vi "Output Processing.vi"(0 "Measurements":T2, 5 "Software Flags":T1, 7 "Powerdown?":bool, 11 "error in (no error)":errorcluster) -> (4 "Measurement Results":T4, 15 "error out":errorcluster)   [LabVIEW 2024, in "devicePowerSequencerCoreLogic.lvlib"]
uses:
  devicePowerSequencerCoreLogic.lvlib
  Measurement Results.ctl
  controls/Measurements.ctl
  controls/Voltage and Current Measurements.ctl
  controls/Software Flags.ctl
  <vilib>/Utility/error.llb/Trim Whitespace One-Sided.vi
  Device Power Sequencer.lvlib
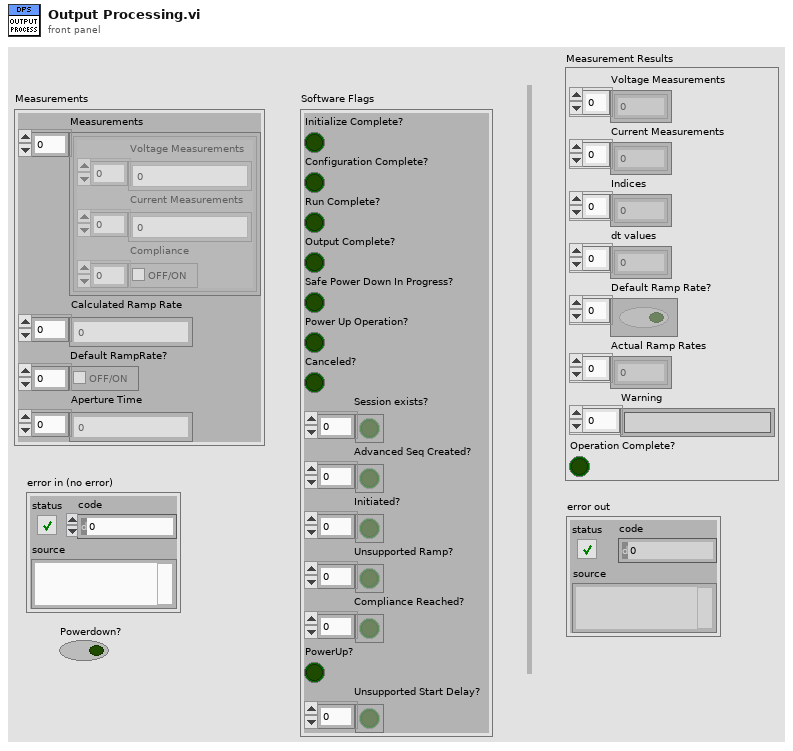
[diagram p1: front panel]
types:
  T1 = typedef "devicePowerSequencerCoreLogic.lvlib/Software Flags.ctl" = cluster{"Initialize Complete?":bool, "Configuration Complete?":bool, "Run Complete?":bool, "Output Complete?":bool, "Safe Power Down In Progress?":bool, "Power Up Operation?":bool, "Canceled?":bool, "Session exists?":bool[], "Advanced Seq Created?":bool[], "Initiated?":bool[], "Unsupported Ramp?":bool[], "Compliance Reached?":bool[], "PowerUp?":bool, "Unsupported Start Delay?":bool[]}
  T2 = typedef "devicePowerSequencerCoreLogic.lvlib/Measurements.ctl" = cluster{"Measurements":T3[], "Calculated Ramp Rate":dbl[], "Default RampRate?":bool[], "Aperture Time":dbl[]}
  T3 = typedef "devicePowerSequencerCoreLogic.lvlib/Voltage and Current Measurements.ctl" = cluster{"Voltage Measurements":dbl[], "Current Measurements":dbl[], "Compliance":bool[]}
  T4 = typedef "Device Power Sequencer.lvlib/Measurement Results.ctl" = cluster{"Voltage Measurements":dbl[], "Current Measurements":dbl[], "Indices":i32[], "dt values":dbl[], "Default Ramp Rate?":bool[], "Actual Ramp Rates":dbl[], "Warning":string[], "Operation Complete?":bool}
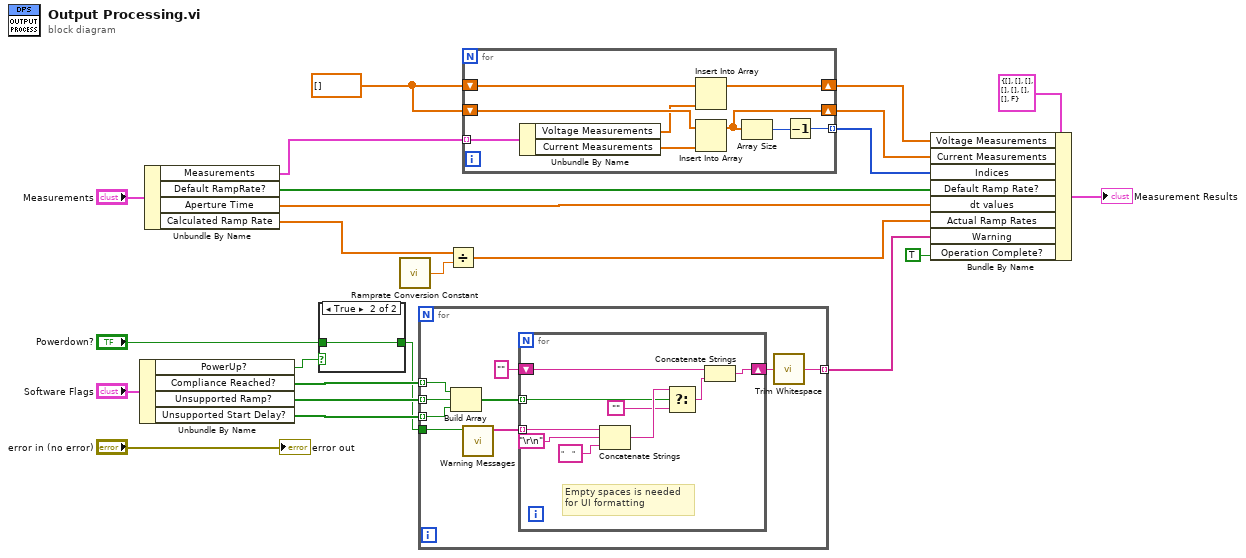
[diagram p0: block diagram]
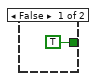
[diagram p2: hidden frame]
diagram:
  w23 = dbl[] []
  n1 = Unbundle By Name("Software Flags") -> ("PowerUp?"=w4:bool, "Compliance Reached?"=w14:bool[], "Unsupported Ramp?"=w13:bool[], "Unsupported Start Delay?"=w5:bool[])
  n2 = Unbundle By Name("Measurements") -> ("Measurements"=w6:T3[], "Default RampRate?"=w18:bool[], "Aperture Time"=w16:dbl[], "Calculated Ramp Rate"=w10:dbl[])
  n3 = case shown="True" w4 {
    tunnel: [TRUE ("Power Down") w25] -> w2
    tunnel: "Powerdown?" -> [_ w25]
    frame False {
    }
    frame True {
    }
  }
  n4 = call "Ramprate Conversion Constant.vi"() -> ("ramp rate conversion constant"=w11:dbl)  [unwired: 15 in]
  n5 = for {
    tunnel: w14 -> [w34] mode=indexing
    tunnel: w13 -> [w33] mode=indexing
    tunnel: [w27] -> w8 mode=indexing
    tunnel: w5 -> [w32] mode=indexing
    tunnel: w2 -> [w26]
    n6 = Build Array(w34, w33, w32) -> (w31:bool[])
    n7 = call "Warning Messages.vi"("Powerdown?"=w26) -> ("Warning Messages"=w28:string[])  [unwired: 10 in]
    n8 = for {
      tunnel: w31 -> [w35] mode=indexing
      shift-right: [w42] -> w29
      shift-left: "" -> [w43]
      tunnel: w28 -> [w41] mode=indexing
      # "Empty spaces is needed \nfor UI formatting"
      n9 = Concatenate Strings(w41, "\r\n", "    " ("string")) -> (w39:string)
      n10 = Select(t=w39, s=w35, f="") -> (s? t:f=w38:string)
      n11 = Concatenate Strings(w43, w38) -> (w42:string)
    }
    n12 = call <vilib>:"Trim Whitespace.vi"("string"=w29) -> ("trimmed string"=w27:string)  [unwired: 1 in]
  }
  n13 = Divide(x=w10, y=w11) -> (x/y=w9:dbl[])
  n14 = for {
    tunnel: w6 -> [w46] mode=indexing
    shift-right: [w50] -> w21
    shift-left: w23 -> [w52]
    shift-right: [w49] -> w20
    shift-left: w23 -> [w51]
    tunnel: [w47] -> w19 mode=indexing
    n15 = Unbundle By Name(w46) -> ("Voltage Measurements"=w45:dbl[], "Current Measurements"=w44:dbl[])
    n16 = Insert Into Array(array=w52, new element=w45) -> (w50:dbl[])  [unwired: 1 in]
    n17 = Insert Into Array(array=w51, new element=w44) -> (w49:dbl[])  [unwired: 1 in]
    n18 = Array Size(array=w49) -> (size(s)=w48:i32)
    n19 = Decrement(x=w48) -> (x-1=w47:i32)
  }
  n20 = Bundle By Name(cluster=T4 {"Voltage Measurements"=[], "Current Measurements"=[], "Indices"=[], "dt values"=[], "Default Ramp Rate?"=[], "Actual Ramp Rates"=[], "Warning"=[], "Operation Complete?"=FALSE} ("Measurement Results"), "Voltage Measurements"=w21, "Current Measurements"=w20, "Indices"=w19, "Default Ramp Rate?"=w18, "dt values"=w16, "Actual Ramp Rates"=w9, "Warning"=w8, "Operation Complete?"=TRUE) -> (→"Measurement Results":T4)
  "error out" <- "error in (no error)"
